vi "GetPiece.vi"(8 "error in (no error)":errorcluster, 11 "Piece in":refnum<class "Piece.lvclass">) -> (0 "error out":errorcluster, 1 "pieceDrawing":T2, 2 "piece":T3, 3 "Piece out":refnum<class "Piece.lvclass">, 4 "color":T1)   [LabVIEW 2020, in "Piece.lvclass"]
uses:
  Piece.lvclass
  typedefs/pieceType.ctl
  <vilib>/picture/picture.llb/imagedata.ctl
  typedefs/pieceColor.ctl
  Piece.lvclass/Piece.ctl
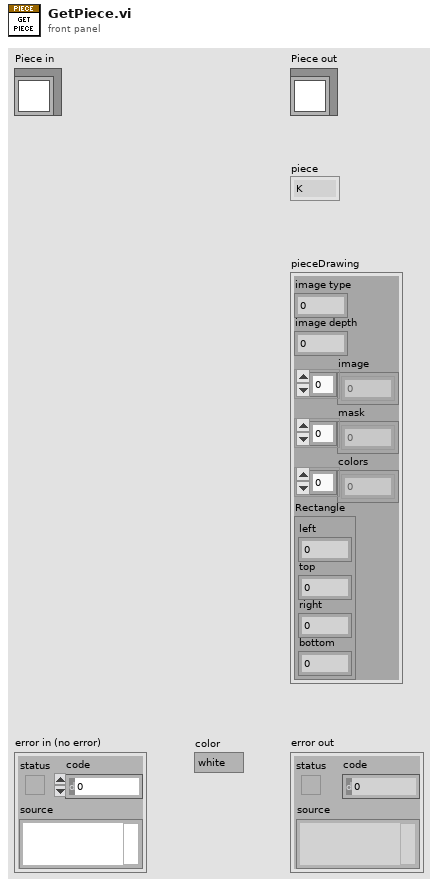
[diagram p1: front panel]
types:
  T1 = typedef "Piece.lvclass/pieceColor.ctl" = enum16{"white", "black"}
  T2 = typedef "imagedata.ctl" = cluster{"image type":i32, "image depth":i32, "image":u8[], "mask":u8[], "colors":u32[], "Rectangle":cluster{"left":i16, "top":i16, "right":i16, "bottom":i16}}
  T3 = typedef "Piece.lvclass/pieceType.ctl" = enum16{"K", "Q", "R", "N", "B", "P", "none"}
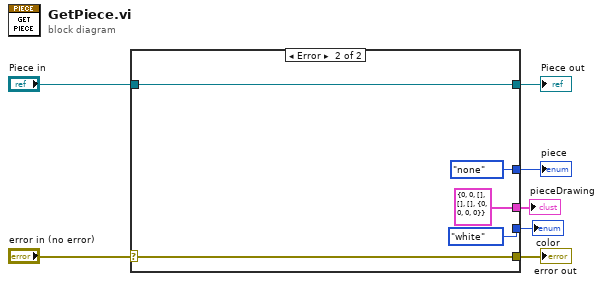
[diagram p0: block diagram]
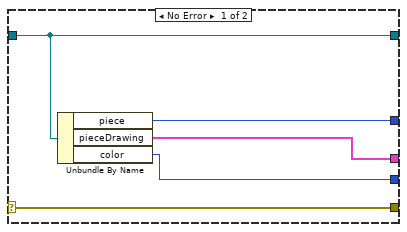
[diagram p2: hidden frame]
diagram:
  n1 = case shown="Error" "error in (no error)" {
    selector: "error in (no error)" -> [w12 w16]
    tunnel: [w12 w16] -> w6
    tunnel: [w11 w17] -> w4
    tunnel: "Piece in" -> [w11 w17]
    tunnel: [w10 pieceType."none" ("piece")] -> w3
    tunnel: [w9 T2 {"image type"=0, "image depth"=0, "image"=[], "mask"=[], "colors"=[], "Rectangle"={"left"=0, "top"=0, "right"=0, "bottom"=0}} ("pieceDrawing")] -> w2
    tunnel: [w8 pieceColor."white" ("color")] -> w1
    frame No Error {
      n2 = Unbundle By Name(w11) -> ("piece"=w10:T3, "pieceDrawing"=w9:T2, "color"=w8:T1)
    }
    frame Error {
    }
  }
  "error out" <- w6
  "Piece out" <- w4
  "piece" <- w3
  "pieceDrawing" <- w2
  "color" <- w1
